vi "_FPGA_Aux_SinusoidalWfmOutput.vi"(0 "DeCycle_U32":u32, 5 "Start strobe":bool, 7 "Beta*2^31_U32":u32, 9 "Parameter1":u64, 11 "Parameter2":u64=1, 13 "Init strobe":bool) -> (4 "AuxVoltage":fxp<+/-,16,14>)   [LabVIEW 2018]
uses:
  <instrlib>/_niInstr/Basic Elements/v1/FPGA/niInstr Basic Elements v1 FPGA.lvlib
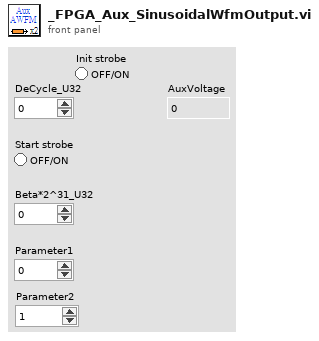
[diagram p1: front panel]
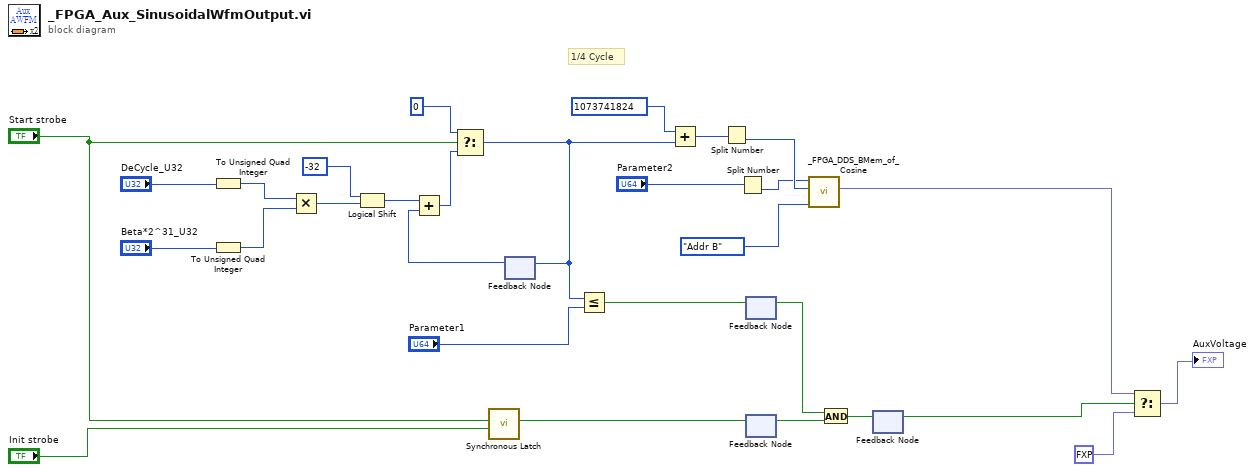
[diagram p0: block diagram]
diagram:
  # "1/4 Cycle"
  n1 = To Unsigned Quad Integer(1:"DeCycle_U32") -> (0:w23:u64)
  n2 = To Unsigned Quad Integer(1:"Beta*2^31_U32") -> (0:w21:u64)
  n3 = Multiply(x=w23, y=w21) -> (x*y=w29:u64)
  n4 = Logical Shift(y=i16 -32, x=w29) -> (x << y=w20:u64)
  n5 = call <instrlib>:"Synchronous Latch.vi"("clear"="Init strobe", "set"="Start strobe") -> ("out"=w26:bool)  [unwired: 9 in]
  n6 = feedback #1() -> (w9:u64)  [unwired: 1 in]
  n7 = Add(x=w20, y=w9) -> (x+y=w17:u64)
  n8 = Select(t=u64 0, s="Start strobe", f=w17) -> (s? t:f=w6:u64)
  n9 = feedback-in #1(w6) -> ()
  n10 = Less Or Equal?(x=w6, y="Parameter1") -> (x <= y?=w12:bool)
  n11 = Add(x=u64 1073741824 ("t"), y=w6) -> (x+y=w5:u64)
  n12 = Split Number(x=w5) -> (lo(x)=w8:u32)  [unwired: 1 out]
  n13 = Split Number(x="Parameter2") -> (lo(x)=w2:u32)  [unwired: 1 out]
  n14 = feedback-in #2(w12) -> ()
  n15 = feedback #2() -> (w3:bool)  [unwired: 1 in]
  n16 = feedback-in #3(w26) -> ()
  n17 = feedback #3() -> (w15:bool)  [unwired: 1 in]
  n18 = call "_FPGA_DDS_BMem_of_Cosine.vi"("Addr"=enum16{"Addr A", "Addr B"}."Addr B", "Cycle_in"=w8, "NormAmp*2^29"=w2) -> ("cos"=w7:fxp<+/-,16,14>)  [unwired: 8 in]
  n19 = And(x=w3, y=w15) -> (x .and. y?=w13:bool)
  n20 = feedback #4() -> (w14:bool)  [unwired: 1 in]
  n21 = feedback-in #4(w13) -> ()
  n22 = Select(t=w7, s=w14, f=fxp<+/-,16,14> 0.0) -> (s? t:f=→"AuxVoltage":fxp<+/-,16,14>)
